vi "FTW-CodeGen-Image.vi"(0 "State In":T1 {"Actor Interface"."Bounds"."Left" format="%dpx"; "Actor Interface"."Bounds"."Top" format="%dpx"; "Actor Interface"."Bounds"."Right" format="%dpx"; "Actor Interface"."Bounds"."Bottom" format="%dpx"}, 5 "XRef":refnum<vi>) -> (4 "Image":picture)   [LabVIEW 2015, in "FTW-Actor-Spawn.xnode"]
uses:
  FTW-Actor-Spawn.xnode
  FTW-CodeGen-State.ctl
panel:
  # "Inputs"
  # "Outputs"
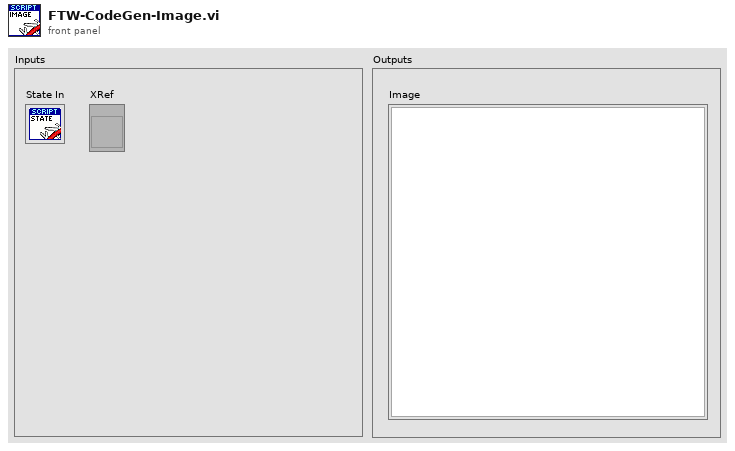
[diagram p1: front panel]
types:
  T1 = typedef "FTW-Actor-Spawn.xnode/FTW-CodeGen-State.ctl" = cluster{"Path Wired?":bool, "Actor Interface":cluster{"Name":string, "Type":variant, "Bounds":cluster{"Left":i32, "Top":i32, "Right":i32, "Bottom":i32}, "Input":bool, "Recommended":bool, "Required":bool, "Dynamic Dispatch":bool, "On Interface":bool, "\"The\" Config Terminal":bool}[], "Config Terminal Index":i32}
  T2 = cluster{"Wired?":bool, "Input?":bool, "\"The\" Actor Configuration":bool, "Type":variant, "Bounds":cluster{"Left":i32, "Top":i32, "Right":i32, "Bottom":i32}}[]
  T3 = cluster{"Left":i32, "Top":i32, "Right":i32, "Bottom":i32}
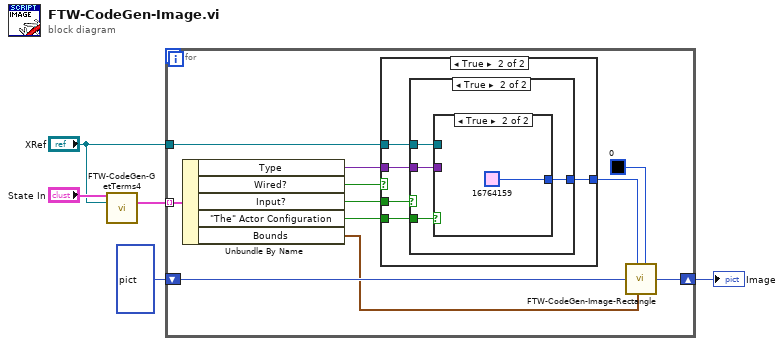
[diagram p0: block diagram]
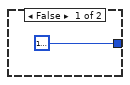
[diagram p2: hidden frame]
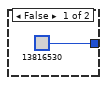
[diagram p3: hidden frame]
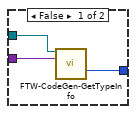
[diagram p4: hidden frame]
diagram:
  n1 = call "FTW-CodeGen-GetTerms4.vi"("State In"="State In", "XRef"="XRef") -> ("Actor Terminals"=w2:T2)  [unwired: 12 in, 1 out]
  n2 = for {
    shift-right: [w15] -> w5
    shift-left: picture bytes[7986] ("Image") -> [w16]
    tunnel: w2 -> [w13] mode=indexing
    tunnel: "XRef" -> [w12]
    n3 = Unbundle By Name(w13) -> ("Type"=w11:variant, "Wired?"=w8:bool, "Input?"=w7:bool, "\"The\" Actor Configuration"=w6:bool, "Bounds"=w14:T3)
    n4 = case shown="True" w8 {
      tunnel: w12 -> [_ w22]
      tunnel: w11 -> [_ w21]
      tunnel: [u32 16777216 ("Border Color") w20] -> w9
      tunnel: w7 -> [_ w19]
      tunnel: w6 -> [_ w18]
      frame False {
      }
      frame True {
        n5 = case shown="True" w19 {
          tunnel: w22 -> [_ w27]
          tunnel: w21 -> [_ w26]
          tunnel: [u32 13816530 ("Border Color") w25] -> w20
          tunnel: w18 -> [_ w24]
          frame False {
          }
          frame True {
            n6 = case shown="True" w24 {
              tunnel: w27 -> [w30 _]
              tunnel: w26 -> [w29 _]
              tunnel: [w28 u32 16764159 ("Border Color")] -> w25
              frame False {
                n7 = call "FTW-CodeGen-GetTypeInfo.vi"("XRef"=w30, "Type Information In"=w29) -> ("Data Type Color"=w28:u32)  [unwired: 10 in, 3 out]
              }
              frame True {
              }
            }
          }
        }
      }
    }
    n8 = call "FTW-CodeGen-Image-Rectangle.vi"("Fill Color"=w9, "Initial Picture"=w16, "Rectangle"=w14, "Border Color"=u32 0) -> ("Picture"=w15:picture)  [unwired: 5 in]
  }
  "Image" <- w5
